vi "获取时间.vi"() -> (0 "当前秒":string, 3 "当前小时数":string, 8 "当前时间":string, 11 "当前日期":string)   [LabVIEW 2016]
uses:
  <vilib>/regexp/Match Regular Expression.xnode
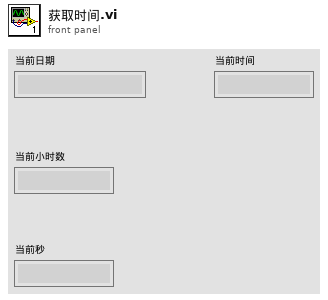
[diagram p1: front panel]
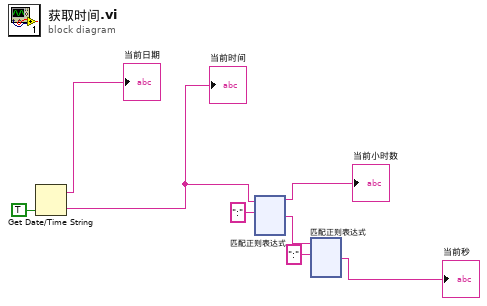
[diagram p0: block diagram]
diagram:
  n1 = Get Date/Time String(want seconds? (F)=TRUE ("需要秒？(F)")) -> (date string=→"当前日期":string, time string=w6:string)  [unwired: 2 in]
  "当前时间" <- w6
  n2 = xnode "匹配正则表达式"("输入字符串"=w6, "正则表达式"=":") -> ("匹配之前"=→"当前小时数":string, "匹配之后"=w3:string)  [unwired: 4 in, 3 out]
  n3 = xnode "匹配正则表达式"("输入字符串"=w3, "正则表达式"=":") -> ("匹配之后"=→"当前秒":string)  [unwired: 4 in, 4 out]
